vi "Test ESPN SQL DB.vi"() -> ()   [LabVIEW 2013]
uses:
  Controls/ALTS-2015 Serial DB Details.ctl
  Controls/ALTS-2015 DB Driver Options.ctl
panel:
  out "error out":errorcluster
  out "Serial Details from DB":T1
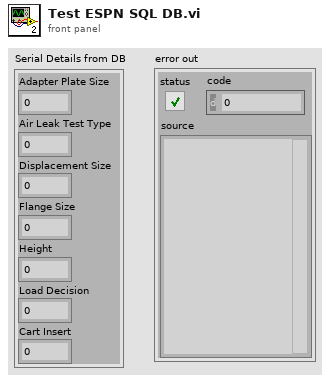
[diagram p1: front panel]
types:
  T1 = typedef "ALTS-2015 Serial DB Details.ctl" = cluster{"Adapter Plate Size":i32, "Air Leak Test Type ":i32, "Displacement Size":i32, "Flange Size":i32, "Height":i32, "Load Decision":i32, "Cart Insert":i32}
  T2 = typedef "ALTS-2015 DB Driver Options.ctl" = enum16{"Init", "Read DB", "Close"}
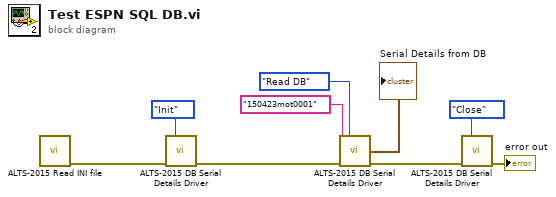
[diagram p0: block diagram]
diagram:
  n1 = call "ALTS-2015 Read INI file.vi"() -> ("error out"=w2:errorcluster)  [unwired: 11 in]
  n2 = call "ALTS-2015 DB Serial Details Driver.vi"("Operation"=ALTS-2015_DB_Driver_Options."Init", "error in (no error)"=w2) -> ("error out"=w5:errorcluster)  [unwired: 11 in, 2 out]
  n3 = call "ALTS-2015 DB Serial Details Driver.vi"("Serial Number"="150423mot0001", "Operation"=ALTS-2015_DB_Driver_Options."Read DB", "error in (no error)"=w5) -> ("Serial Details from DB"=→"Serial Details from DB":T1, "error out"=w6:errorcluster)  [unwired: 10 in, 1 out]
  n4 = call "ALTS-2015 DB Serial Details Driver.vi"("Operation"=ALTS-2015_DB_Driver_Options."Close", "error in (no error)"=w6) -> ("error out"=→"error out":errorcluster)  [unwired: 11 in, 2 out]
